vi "浮点数所在区间（利用阙值插值）.vi"(1 "比较值":dbl, 2 "阙值数组":dbl[](array[numeric])) -> (0 "区间索引":i32)   [LabVIEW 2012]
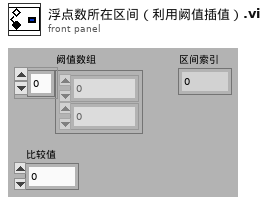
[diagram p1: front panel]
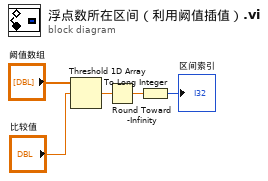
[diagram p0: block diagram]
diagram:
  n1 = Threshold 1D Array(2:"比较值", 3:"阙值数组") -> (0:w3:dbl)  [unwired: 1 in]
  n2 = Round Toward -Infinity(1:w3) -> (0:w2:dbl)
  n3 = To Long Integer(number=w2) -> (32bit integer=→"区间索引":i32)
